vi "G-Audio - IEEE Float Compare.vi"() -> ()   [LabVIEW 2020]
doc: "An example comparing lossless / lossy writing and reading of 32-bit IEEE Float (SGL) WAV files."
uses:
  <vilib>/sound2/lvsound2.llb/Sound Data Format.ctl
  G-Audio/Controls/Audio File Info.ctl
  G-Audio/Controls/WAV Codec Specific Info.ctl
  G-Audio/Controls/WAV Container Format.ctl
  G-Audio/Controls/WAV Data Format.ctl
  <vilib>/Utility/sysdir.llb/System Directory Type.ctl
  G-Audio/Polymorphic VIs/Open Audio File Write (WAV).vi
  45e09a5f-307f-4719-b7dc-40eb757bf721.vi
  ebf7a747-ff34-43af-a363-791bc307e7e5.vi
  G-Audio/Private/Get Codec.vi
  G-Audio/Private/Result To Error.vi
  45e09a5f-307f-4719-b7dc-40eb757bf721.vi/fba40667-3e21-44fa-934c-95909d78721c.vi
  G-Audio/Private/Get Basic Audio File Info.vi
  ebf7a747-ff34-43af-a363-791bc307e7e5.vi/779dfdfd-1b42-4cf4-8001-66d3dd167625.vi
  ebf7a747-ff34-43af-a363-791bc307e7e5.vi/55d550d4-9624-414e-aebd-6e02b5081896.vi
  G-Audio/Private/Get File Extension (Reentrant).vi
  45e09a5f-307f-4719-b7dc-40eb757bf721.vi/fba40667-3e21-44fa-934c-95909d78721c.vi/4b7b629c-2e91-4160-9820-a26af8f6e677.vi
  45e09a5f-307f-4719-b7dc-40eb757bf721.vi/fba40667-3e21-44fa-934c-95909d78721c.vi/e7c4a249-ce38-42b4-8985-5fdb76b4ebfc.vi
  ebf7a747-ff34-43af-a363-791bc307e7e5.vi/779dfdfd-1b42-4cf4-8001-66d3dd167625.vi/a9d2058a-38f9-4c88-a1a9-9bf864ebbde5.vi
  ebf7a747-ff34-43af-a363-791bc307e7e5.vi/55d550d4-9624-414e-aebd-6e02b5081896.vi/4b7b629c-2e91-4160-9820-a26af8f6e677.vi
  ebf7a747-ff34-43af-a363-791bc307e7e5.vi/55d550d4-9624-414e-aebd-6e02b5081896.vi/e7c4a249-ce38-42b4-8985-5fdb76b4ebfc.vi
  <vilib>/Utility/error.llb/Error Cluster From Error Code.vi
  <vilib>/sound2/lvsound2.llb/Sound File Write Open.vi
  <vilib>/sound2/lvsound2.llb/Sound File Write (SGL).vi
  <vilib>/sound2/lvsound2.llb/Sound File Info (path).vi
  <vilib>/sound2/lvsound2.llb/Sound File Read Open.vi
  <vilib>/sound2/lvsound2.llb/Sound File Read (SGL).vi
  <vilib>/Utility/Data Type/Get Numeric Information.vi
  <vilib>/measure/NI_MABase.lvlib
  G-Audio/G-Audio.lvlib
panel:
  out "G-Audio Error":errorcluster
  out "LabVIEW Sound Error":errorcluster
  out "LabVIEW Sound Equal?":bool
  out "G-Audio Equal?":bool
  # "This VI writes 32-bit IEEE Float WAV files using LabVIEW Sound and G-Audio, then reads and compares them with the original data. Audio data should be identical."
  # "G"
  # "-Audio"
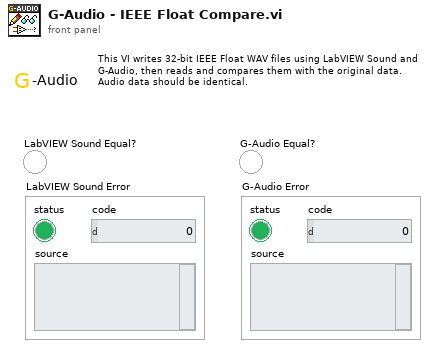
[diagram p1: front panel]
types:
  T1 = typedef "System Directory Type.ctl" = i32
  T2 = typedef "G-Audio.lvlib/WAV Codec Specific Info.ctl" = cluster{"Container Format":T3, "Data Format":T4}
  T3 = typedef "G-Audio.lvlib/WAV Container Format.ctl" = enum32{"RIFF", "Wave64"}
  T4 = typedef "G-Audio.lvlib/WAV Data Format.ctl" = u32
  T5 = typedef "G-Audio.lvlib/Audio File Info.ctl" = cluster{"Sample Rate (Hz)":u32, "Channels":u32, "Bit Depth":u32}
  T6 = typedef "Sound Data Format.ctl" = cluster{"sample rate (S/s)":dbl, "number of channels":i32, "bits per sample":i32}
  T7 = typedef "Sound File Refnum.ctl" = refnum<file>
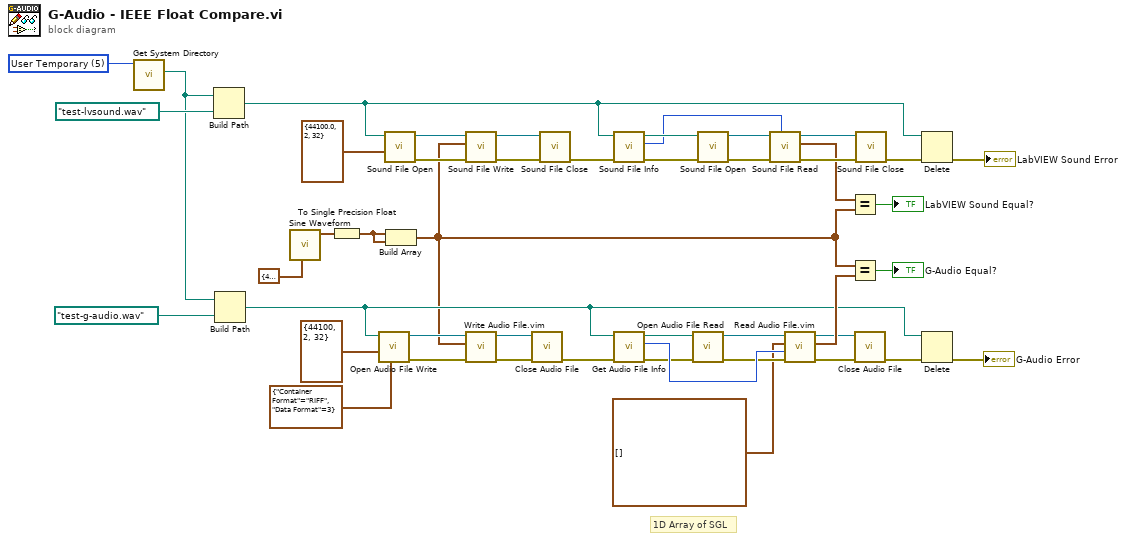
[diagram p0: block diagram]
diagram:
  w19 = T1 5 items=["User Home"=0, "User Desktop"=1, "User Documents"=2, "User Application Data"=3, "User Preferences"=4, "User Temporary"=5, "Public Documents"=6, "Public Application Data"=7, "Public Preferences"=8, "Public Cache"=13, "System Core Libraries"=9, "System Installed Libraries"=10, "Application Files"=11, "Boot Volume Root"=12] ("system directory type")
  # "1D Array of SGL"
  n1 = call <vilib>:"Get System Directory.vi"("system directory type"=w19) -> ("system directory"=w17:path)  [unwired: 10 in]
  n2 = Build Path(base path=w17, name or relative path=path "test-lvsound.wav" ("path")) -> (appended path=w5:path)
  n3 = Build Path(base path=w17, name or relative path=path "test-g-audio.wav" ("path")) -> (appended path=w15:path)
  n4 = call <vilib>:"Sine Waveform.vi"("sampling info"=cluster{"Fs":dbl, "#s":dbl} {"Fs"=44100.0, "#s"=44100.0}) -> ("signal out"=w44:waveform(dbl))  [unwired: 9 in, 1 out]
  n5 = To Single Precision Float(number=w44) -> (single precision float=w3:waveform(sgl))
  n6 = call-poly "Open Audio File Write.vi"("Codec Specific Info"=T2 {"Container Format"=enum."RIFF", "Data Format"=3}, "Audio File Info"=T5 {"Sample Rate (Hz)"=44100, "Channels"=2, "Bit Depth"=32}, "Path"=w15) -> ("error out"=w30:errorcluster, "Audio File Refnum"=w32:refnum<file>)  [unwired: 7 in]
  n7 = call-poly <vilib>:"Sound File Open.vi"("sound format"=T6 {"sample rate (S/s)"=44100.0, "number of channels"=2, "bits per sample"=32}, "path"=w5) -> ("error out"=w41:errorcluster, "sound file refnum"=w43:T7)  [unwired: 8 in]
  n8 = Build Array(w3, w3) -> (w4:waveform(sgl)[])
  n9 = call-poly <vilib>:"Sound File Write.vi"("error in (no error)"=w41, "data"=w4, "sound file refnum"=w43) -> ("error out"=w40:errorcluster, "sound file refnum out"=w42:T7)  [unwired: 7 in]
  n10 = call "Write Audio File.vim"("error in (no error)"=w30, "Audio Data"=w4, "Audio File Refnum In"=w32) -> ("error out"=w29:errorcluster, "Audio File Refnum Out"=w31:refnum<file>)  [unwired: 7 in]
  n11 = call "Close Audio File.vi"("error in (no error)"=w29, "Audio File Refnum In"=w31) -> ("error out"=w28:errorcluster)  [unwired: 9 in]
  n12 = call <vilib>:"Sound File Close.vi"("error in (no error)"=w40, "sound file refnum"=w42) -> ("error out"=w25:errorcluster)  [unwired: 9 in]
  n13 = call-poly <vilib>:"Sound File Info.vi"("error in (no error)"=w25, "path"=w5) -> ("error out"=w24:errorcluster, "total number of samples/ch"=w22:u32, "path out"=w23:path)  [unwired: 6 in, 1 out]
  n14 = call "Get Audio File Info.vi"("error in (no error)"=w28, "Path In"=w15) -> ("error out"=w10:errorcluster, "Sample Length"=w12:u64, "Path Out"=w13:path)  [unwired: 6 in, 1 out]
  n15 = call "Open Audio File Read.vi"("error in (no error)"=w10, "Path"=w13) -> ("error out"=w8:errorcluster, "Audio File Refnum"=w14:refnum<file>)  [unwired: 8 in]
  n16 = call-poly <vilib>:"Sound File Open.vi"("error in (no error)"=w24, "path"=w23) -> ("error out"=w38:errorcluster, "sound file refnum"=w39:T7)  [unwired: 8 in]
  n17 = call-poly <vilib>:"Sound File Read.vi"("number of samples/ch (-1: all)"=w22, "error in (no error)"=w38, "sound file refnum"=w39) -> ("error out"=w37:errorcluster, "data"=w21:waveform(sgl)[], "sound file refnum out"=w36:T7)  [unwired: 4 in, 2 out]
  n18 = call "Read Audio File.vim"("error in (no error)"=w8, "Samples To Read"=w12, "Data Format"=waveform(sgl)[] [], "Audio File Refnum In"=w14) -> ("error out"=w9:errorcluster, "Audio Data"=w26:waveform(sgl)[], "Audio File Refnum Out"=w11:refnum<file>)  [unwired: 3 in, 2 out]
  n19 = Equal?(x=w21, y=w4) -> (x = y?=→"LabVIEW Sound Equal?":bool)
  n20 = Equal?(x=w4, y=w26) -> (x = y?=→"G-Audio Equal?":bool)
  n21 = call "Close Audio File.vi"("error in (no error)"=w9, "Audio File Refnum In"=w11) -> ("error out"=w7:errorcluster)  [unwired: 9 in]
  n22 = call <vilib>:"Sound File Close.vi"("error in (no error)"=w37, "sound file refnum"=w36) -> ("error out"=w35:errorcluster)  [unwired: 9 in]
  n23 = Delete(path (use dialog)=w5, error in=w35) -> (error out=→"LabVIEW Sound Error":errorcluster)  [unwired: 3 in, 2 out]
  n24 = Delete(path (use dialog)=w15, error in=w7) -> (error out=→"G-Audio Error":errorcluster)  [unwired: 3 in, 2 out]
